vi "Enter Leonardo Bootloader.vi"(8 "Error In":errorcluster, 11 "VISA resource name":refnum<visa-resource-name>) -> (0 "Error Out":errorcluster, 2 "Found?":bool, 3 "VISA resource name":refnum<visa-resource-name>)   [LabVIEW 2011, in "LVH-LINX.lvlib"]
uses:
  LVH-LINX.lvlib
  <vilib>/Instr/_visa.llb/VISA Find Search Mode.ctl
  <vilib>/Instr/_visa.llb/VISA Configure Serial Port (Instr).vi
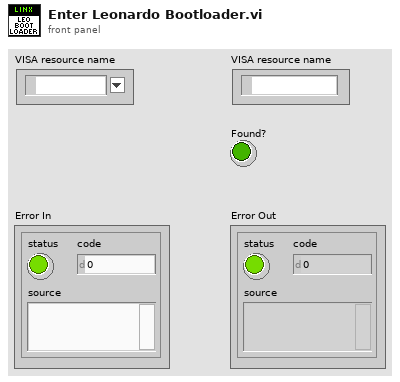
[diagram p1: front panel]
types:
  T1 = typedef "VISA Find Search Mode.ctl" = u32
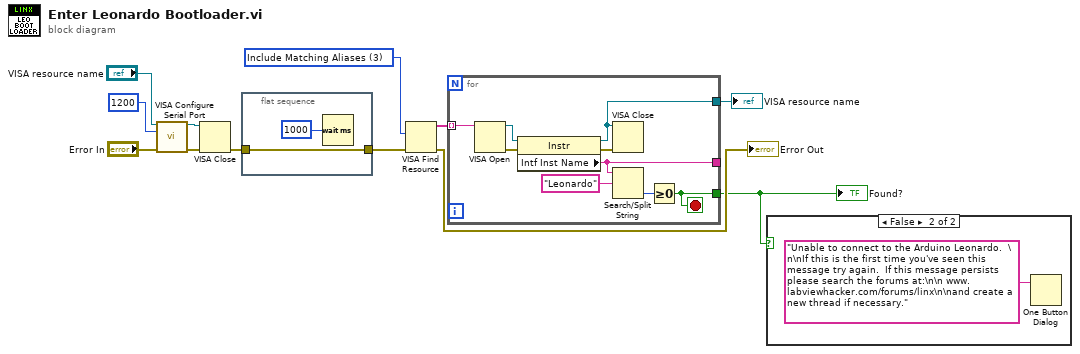
[diagram p0: block diagram]
diagram:
  w12 = T1 3 items=["Canonical Names Only"=0, "Aliases Only"=2, "Include Matching Aliases"=3, "Include All Aliases"=4] ("Search Mode")
  n1 = call-poly "VISA Configure Serial Port"("VISA resource name"="VISA resource name", "baud rate (9600)"=u32 1200, "error in (no error)"="Error In") -> ("VISA resource name out"=w4:refnum<visa-resource-name>, "error out"=w5:errorcluster)  [unwired: 11 in]
  n2 = VISA Close(VISA resource name=w4, error in (no error)=w5) -> (error out=w9:errorcluster)
  n3 = flat-sequence {
    tunnel: [w13] -> w10
    tunnel: w9 -> [w13]
    frame #0 {
      n4 = Wait (ms)(milliseconds to wait=u32 1000) -> ()  [unwired: 1 out]
    }
  }
  n5 = VISA Find Resource(8:w10, 10:w12) -> (0:→"Error Out":errorcluster, 3:w11:string[])  [unwired: 1 in, 1 out]
  n6 = for {
    tunnel: w11 -> [w23] mode=indexing
    tunnel: [w17] -> _
    tunnel: [w16] -> w7
    tunnel: [w15] -> w1
    stop <- w15 stop-if-true
    n7 = VISA Open(VISA resource name=w23) -> (VISA resource name=w22:refnum<visa-resource-name>, error out=w21:errorcluster)  [unwired: 4 in]
    n8 = property class="Instr"(reference=w22, error in=w21) -> (reference out=w16:refnum<visa-resource-name>, error out=w20:errorcluster, "Intf Inst Name"=w17:string)
    n9 = VISA Close(VISA resource name=w16, error in (no error)=w20) -> ()  [unwired: 1 out]
    n10 = Search/Split String(string=w17, search string/char (-)="Leonardo") -> (offset of match=w18:i32)  [unwired: 1 in, 2 out]
    n11 = Greater Or Equal To 0?(x=w18) -> (x >= 0?=w15:bool)
  }
  "Found?" <- w1
  "VISA resource name" <- w7
  n12 = case shown="False" w1 {
    frame True {
    }
    frame False {
      n13 = One Button Dialog(message="Unable to connect to the Arduino Leonardo.  \n\nIf this is the first time you've seen this message try again.  If this message persists please search the forums at:\n\n www.labviewhacker.com/forums/linx\n\nand create a new thread if necessary.") -> ()  [unwired: 1 in, 1 out]
    }
  }
